vi "Read ActionVIs Properties.vi"(8 "error in (no error)":errorcluster, 11 "CustomDeviceRepo in":refnum<class "CustomDeviceRepo.lvclass">) -> (0 "error out":errorcluster, 2 "ActionVIs Properties":T1[](array[typedef]), 3 "CustomDeviceRepo out":refnum<class "CustomDeviceRepo.lvclass">)   [LabVIEW 2014, in "CustomDeviceRepo.lvclass"]
uses:
  CustomDeviceRepo.lvclass
  Custom Device Type Defs/ActionVIs Properties.ctl
  Custom Device XML/Custom Device XML/Path Cluster.ctl
  CustomDeviceRepo.lvclass/CustomDeviceRepo.ctl
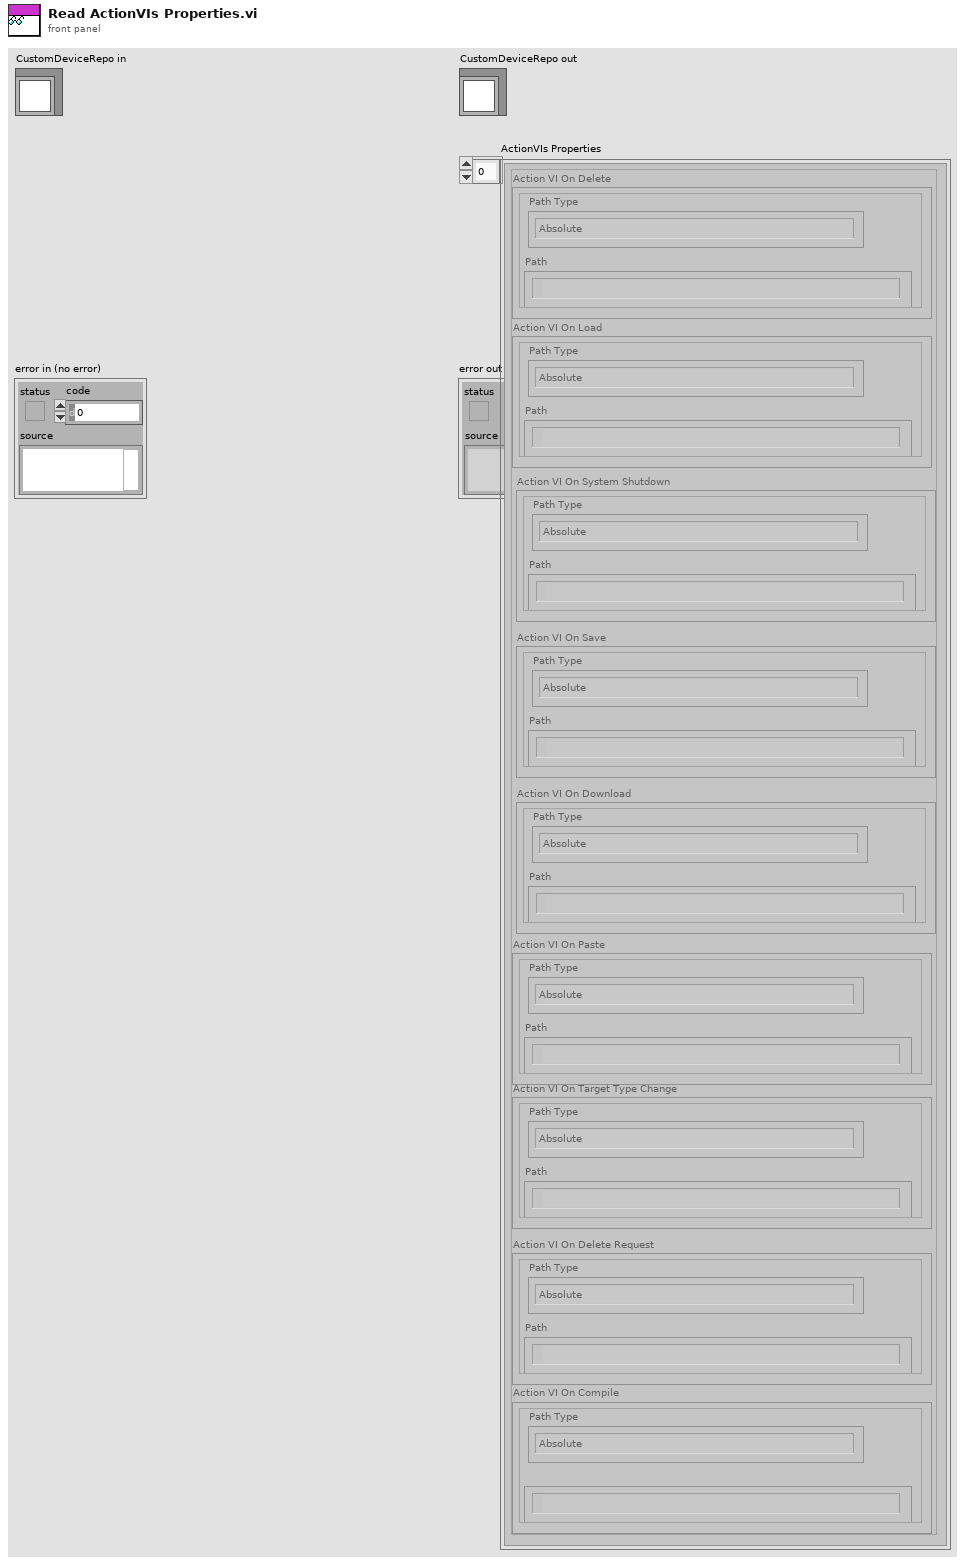
[diagram p1: front panel]
types:
  T1 = typedef "ActionVIs Properties.ctl" = cluster{"Action VI On Delete":T2, "Action VI On Load":T2, "Action VI On Paste":T2, "Action VI On Target Type Change":T2, "Action VI On Delete Request":T2, "Action VI On Compile":T2, "Action VI On System Shutdown":T2, "Action VI On Save":T2, "Action VI On Download":T2}
  T2 = typedef "Path Cluster.ctl" = cluster{"Path":path, "Path Type":enum16{"Absolute", "To Base", "To Common Doc Dir", "To Application Data Dir"}}
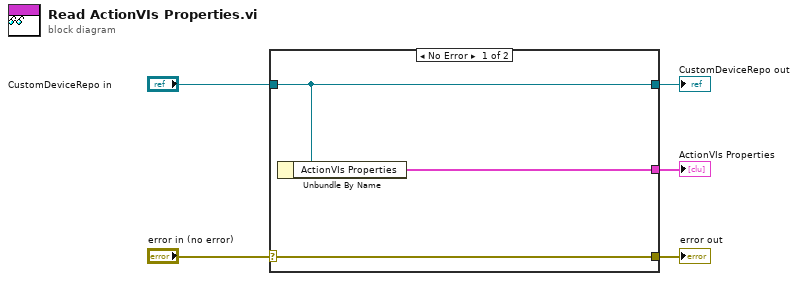
[diagram p0: block diagram]
diagram:
  n1 = case shown="No Error" "error in (no error)" {
    selector: "error in (no error)" -> [w8 w9]
    tunnel: [w8 w9] -> w4
    tunnel: [w7 w10] -> w2
    tunnel: "CustomDeviceRepo in" -> [w7 w10]
    tunnel: [w6 _] -> w1
    frame No Error {
      n2 = Unbundle By Name(w7) -> ("ActionVIs Properties"=w6:T1[])
    }
    frame Error {
    }
  }
  "error out" <- w4
  "CustomDeviceRepo out" <- w2
  "ActionVIs Properties" <- w1
